vi "Check Error.vi"(2 "error in (no error)":errorcluster, 3 "Message":string) -> (0 "error out":errorcluster, 1 "Message Out":string)   [LabVIEW 2014]
doc: "Checks if an error occured in the queue VIs and sets the message to \"Error\"."
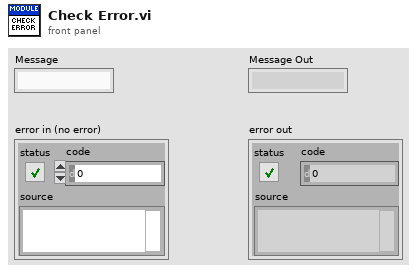
[diagram p1: front panel]
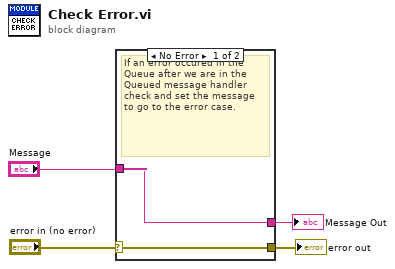
[diagram p0: block diagram]
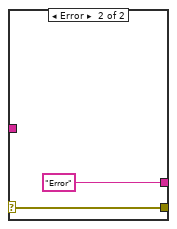
[diagram p2: hidden frame]
diagram:
  n1 = case shown="No Error" "error in (no error)" {
    selector: "error in (no error)" -> [w6 w8]
    tunnel: [w6 w8] -> w4
    tunnel: [w5 "Error" ("y")] -> w3
    tunnel: "Message" -> [w5 _]
    frame No Error {
      # "If an error occured in the Queue after we are in the Queued message handler check and set the message to go to the error case."
    }
    frame Error {
    }
  }
  "error out" <- w4
  "Message Out" <- w3
